vi "Phasor Convert (tau, f) to (m, phi).vi"(1 "Lifetime":dbl[unit], 2 "Phasor Frequency":dbl[unit]) -> (6 "Phasor (m, phi)":T1)   [LabVIEW 2021, in "Phasor.lvlib"]
uses:
  Phasor (m, phi).ctl
  Phasor.lvlib
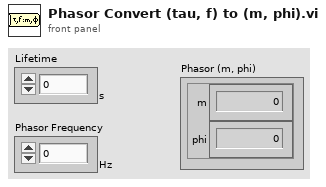
[diagram p1: front panel]
types:
  T1 = typedef "Phasor.lvlib/Phasor (m, phi).ctl" = cluster{"m":dbl, "phi":dbl}
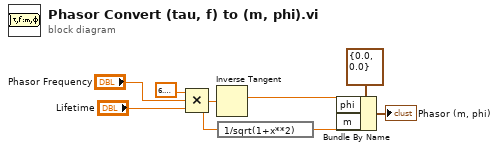
[diagram p0: block diagram]
diagram:
  n1 = Compound Arithmetic op=MULTIPLY(6.283185307179586, "Phasor Frequency", "Lifetime") -> (w5:dbl)
  n2 = Inverse Tangent(1:w5) -> (0:w3:dbl)
  n3 = expression code="1/sqrt(1+x**2)"(w5) -> (w2:dbl)
  n4 = Bundle By Name(cluster=T1 {"m"=0.0, "phi"=0.0} ("Phasor (m, phi)"), "phi"=w3, "m"=w2) -> (→"Phasor (m, phi)":T1)
